vi "Stop TCS.vi"(8 "error in (no error)":errorcluster, 11 "SPARC4_GEI in":refnum<class "SPARC4_GEI.lvclass">) -> (0 "error out":errorcluster, 3 "SPARC4_GEI out":refnum<class "SPARC4_GEI.lvclass">)   [LabVIEW 2018, in "SPARC4_GEI.lvclass"]
uses:
  SPARC4_GEI.lvclass
  SPARC4_GEI.lvclass/SPARC4_GEI.ctl
  TCS/TCS.lvclass
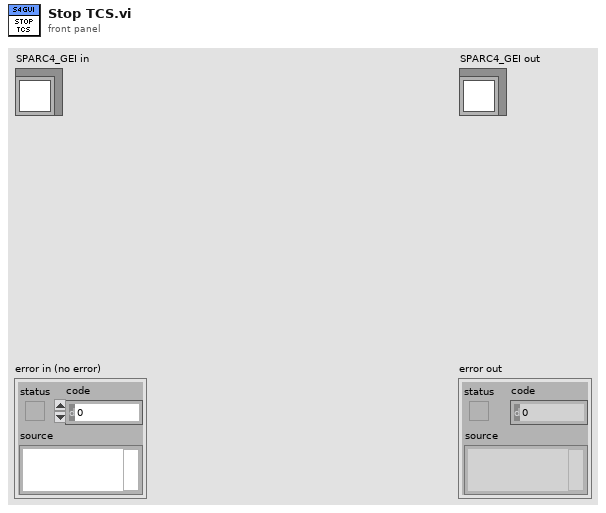
[diagram p1: front panel]
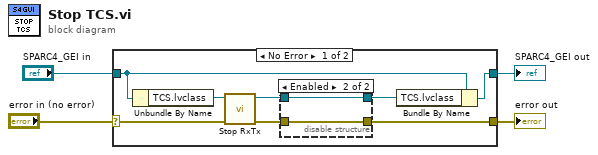
[diagram p0: block diagram]
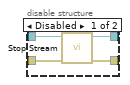
[diagram p2: hidden frame]
diagram:
  n1 = case shown="No Error" "error in (no error)" {
    selector: "error in (no error)" -> [w8 w20]
    tunnel: [w5 w20] -> w3
    tunnel: [w11 w19] -> w1
    tunnel: "SPARC4_GEI in" -> [w12 w19]
    frame No Error {
      n2 = Unbundle By Name(w12) -> ("TCS.lvclass"=w7:refnum<class "TCS.lvclass">)
      n3 = call "Stop RxTx.vi"("error in (no error)"=w8, "TCS in"=w7) -> ("error out"=w10:errorcluster, "TCS out"=w9:refnum<class "TCS.lvclass">)  [unwired: 8 in]
      n4 = disable-structure shown="Enabled" {
        disable-tunnel: w10 -> [w16 w17]
        disable-tunnel: w9 -> [w15 w18]
        disable-tunnel: [w14 w18] -> w6
        disable-tunnel: [w13 w17] -> w5
        frame Disabled {
          n5 = call "Stop Stream.vi"("error in (no error)"=w16, "TCS in"=w15) -> ("error out"=w13:errorcluster, "TCS out"=w14:refnum<class "TCS.lvclass">)  [unwired: 8 in]
        }
        frame Enabled {
        }
      }
      n6 = Bundle By Name(cluster=w12, "TCS.lvclass"=w6) -> (w11:refnum<class "SPARC4_GEI.lvclass">)
    }
    frame Error {
    }
  }
  "error out" <- w3
  "SPARC4_GEI out" <- w1
